vi "Startup.vi"(8 "error in (no error)":errorcluster, 9 "Database":refnum<class "Database.lvclass">, 10 "Config":refnum<class>, 11 "DLP2 in":refnum<class "DLP2.lvclass">) -> (0 "error out":errorcluster, 3 "DLP2 out":refnum<class "DLP2.lvclass">)   [LabVIEW 2022 SP3, in "DLP2.lvclass"]
doc: "Developed by Kevin Thompson\nkevin@thompsonengineering.net\n\nCopyright 2018\nThompson Engineering, LLC"
uses:
  DLP2.lvclass
  Database/Database.lvclass
  DataTypes/Dependency--cluster.ctl
  DLP2.lvclass/DLP2.ctl
  Accessors/Set Dependency.vi
  Accessors/Set VISA Ref.vi
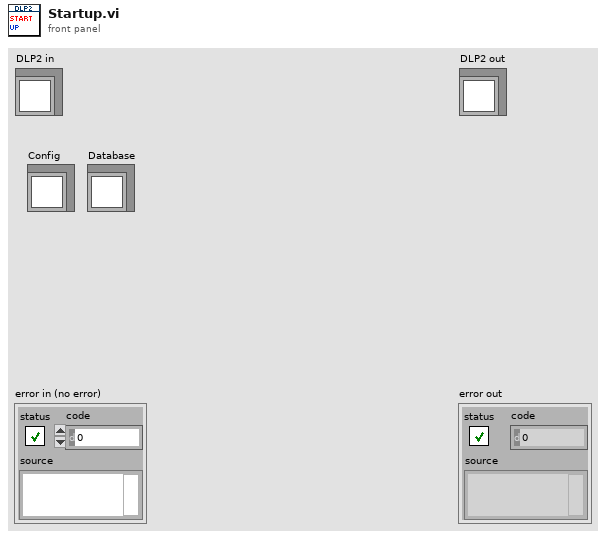
[diagram p1: front panel]
types:
  T1 = typedef "DLP2.lvclass/Dependency--cluster.ctl" = cluster{"Config":refnum<class>, "Database":refnum<class "Database.lvclass">}
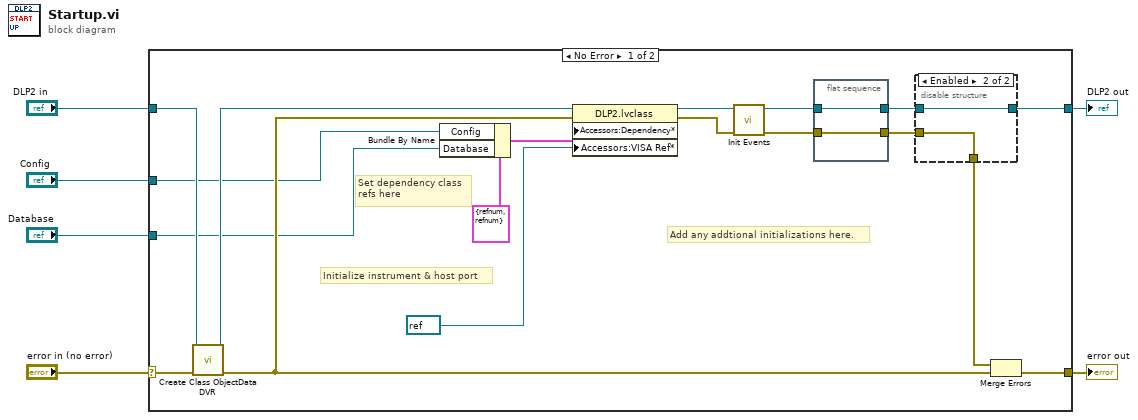
[diagram p0: block diagram]
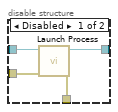
[diagram p2: hidden frame]
diagram:
  n1 = case shown="No Error" "error in (no error)" {
    selector: "error in (no error)" -> [w24 w34]
    tunnel: [w17 w34] -> w5
    tunnel: [w14 w33] -> w3
    tunnel: "DLP2 in" -> [w22 w33]
    tunnel: "Config" -> [w9 _]
    tunnel: "Database" -> [w7 _]
    frame No Error {
      # "Set dependency class\nrefs here"
      # "Initialize instrument & host port"
      # "Add any addtional initializations here."
      n2 = call "Create Class ObjectData DVR.vi"("error in (no error)"=w24, "DLP2 in"=w22) -> ("error out"=w12:errorcluster, "DLP2 out"=w21:refnum<class "DLP2.lvclass">)  [unwired: 8 in]
      n3 = Bundle By Name(cluster=T1 {"Config"=refnum, "Database"=refnum} ("Dependency"), "Config"=w9, "Database"=w7) -> (w8:T1)
      n4 = property class="DLP2.lvclass"(reference=w21, error in=w12, "Accessors:Dependency*"=w8, "Accessors:VISA Ref*"=refnum<visa-resource-name> refnum ("VISA Ref*")) -> (reference out=w23:refnum<class "DLP2.lvclass">, error out=w20:errorcluster)
      n5 = call "Init Events.vi"("error in (no error)"=w20, "DLP2 in"=w23) -> ("error out"=w18:errorcluster, "DLP2 out"=w19:refnum<class "DLP2.lvclass">)  [unwired: 8 in]
      n6 = flat-sequence {
        tunnel: w19 -> [w32]
        tunnel: [w32] -> w15
        tunnel: w18 -> [w31]
        tunnel: [w31] -> w16
        frame #0 {
        }
      }
      n7 = disable-structure shown="Enabled" {
        disable-tunnel: w16 -> [w28 w29]
        disable-tunnel: w15 -> [w27 w30]
        disable-tunnel: [w26 w30] -> w14
        disable-tunnel: [w25 w29] -> w13
        frame Disabled {
          n8 = call "Launch Process.vi"("error in (no error)"=w28, "DLP2 in"=w27) -> ("error out"=w25:errorcluster, "DLP2 out"=w26:refnum<class "DLP2.lvclass">)  [unwired: 6 in, 2 out]
        }
        frame Enabled {
        }
      }
      n9 = Merge Errors(w13, w12) -> (w17:errorcluster)
    }
    frame Error {
    }
  }
  "error out" <- w5
  "DLP2 out" <- w3
